vi "TranReport.vi"(0 "Rings":picture, 1 "3D Surface":refnum<vi>, 2 "annuli list":string[](array[string]), 5 "Output Cluster":T1 {"?" format="%.2f"; "?"."Y[i]=X[i]/Max|X|" format="%.2f"; "?"."output" format="%.2f"; "?" format="%.2f"; "?"."Y[i]=X[i]/Max|X|" format="%.2f"; "?"."?" format="%.2f"}, 7 "Trans Geometry":T2={"Radius (cm)"=9.0, "a (cm)"=4.0, "focus location"=9.0} {"focus location" format="%.2f"; "a (cm)" format="%.2f"; "Radius (cm)" format="%.2f"}, 9 "Center Hole":dbl format="%.2f", 11 "Variables":T3={"Number of rings"=1, "sound spd (cm/s)"=150000, "z span (cm)"=4.0, "z steps"=20, "y spacing (cm)"=0.01, "y steps"=50, "time step (s)"=1e-08, "z"=0.0, "y"=0.0, "ref delay"=0.0, "freq (MHz)"=4.71, "cycles"=300} {"freq (MHz)" format="%.2f"; "z span (cm)" format="%.2f"; "y" format="%.2f"; "ref delay" format="%.2f"; "y spacing (cm)" format="%.3f"; "z" format="%.2f"; "time step (s)" format="%.2e"}, 12 "case":bool, 13 "ring locations":string) -> ()   [LabVIEW 2022 SP3]
uses:
  <vilib>/Utility/NIReport.llb/Append Report Text (str wrap).vi
  <vilib>/Utility/NIReport.llb/NI_report.lvclass
panel:
  out "lateral pressure":cluster{"output":dbl[], "output":dbl[]}(graph)
  out "axial pressure":cluster{dbl[], "output":dbl[]}(graph)
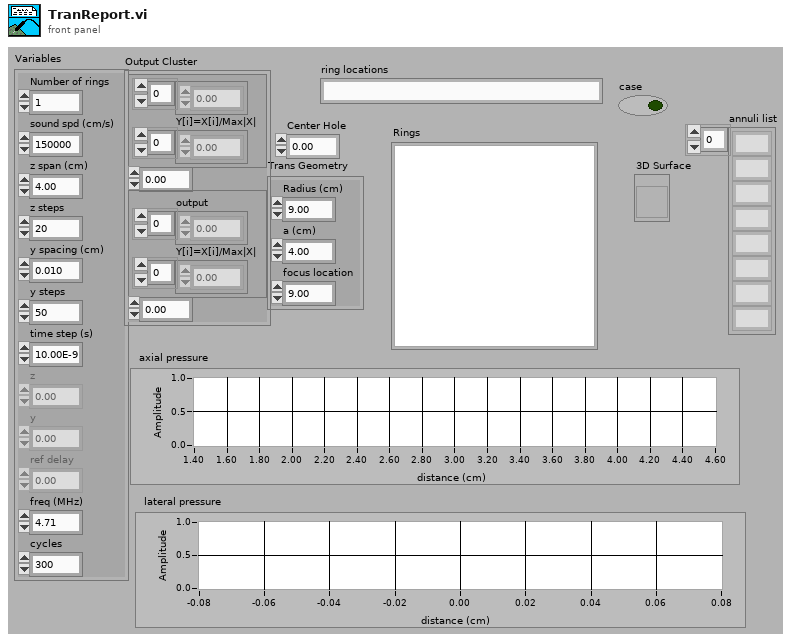
[diagram p1: front panel]
types:
  T1 = cluster{cluster{dbl[], "Y[i]=X[i]/Max|X|":dbl[]}, dbl, cluster{"output":dbl[], "Y[i]=X[i]/Max|X|":dbl[]}, dbl}
  T2 = cluster{"Radius (cm)":dbl, "a (cm)":dbl, "focus location":dbl}
  T3 = cluster{"Number of rings":i32, "sound spd (cm/s)":i32, "z span (cm)":dbl, "z steps":i32, "y spacing (cm)":dbl, "y steps":i32, "time step (s)":sgl, "z":dbl, "y":dbl, "ref delay":dbl, "freq (MHz)":dbl, "cycles":i32}
  T4 = cluster{"top":dbl, "left":dbl, "right":dbl, "bottom":dbl}
  T5 = cluster{"Italic":enum16{"Italic Unchanged", "Italic On", "Italic Off"}, "Strike Through":enum16{"Strike Through Unchanged", "Strike Through On", "Strike Through Off"}, "Underline":enum16{"Underline Unchanged", "Underline On", "Underline Off"}, "Bold":enum16{"Bold Unchanged", "Bold On", "Bold Off"}}
  T6 = cluster{"Charset (-1)":i16, "Weight (-1)":i16, "Name":string, "Size":string}
  T7 = cluster{"output":dbl[], "Y[i]=X[i]/Max|X|":dbl[]}
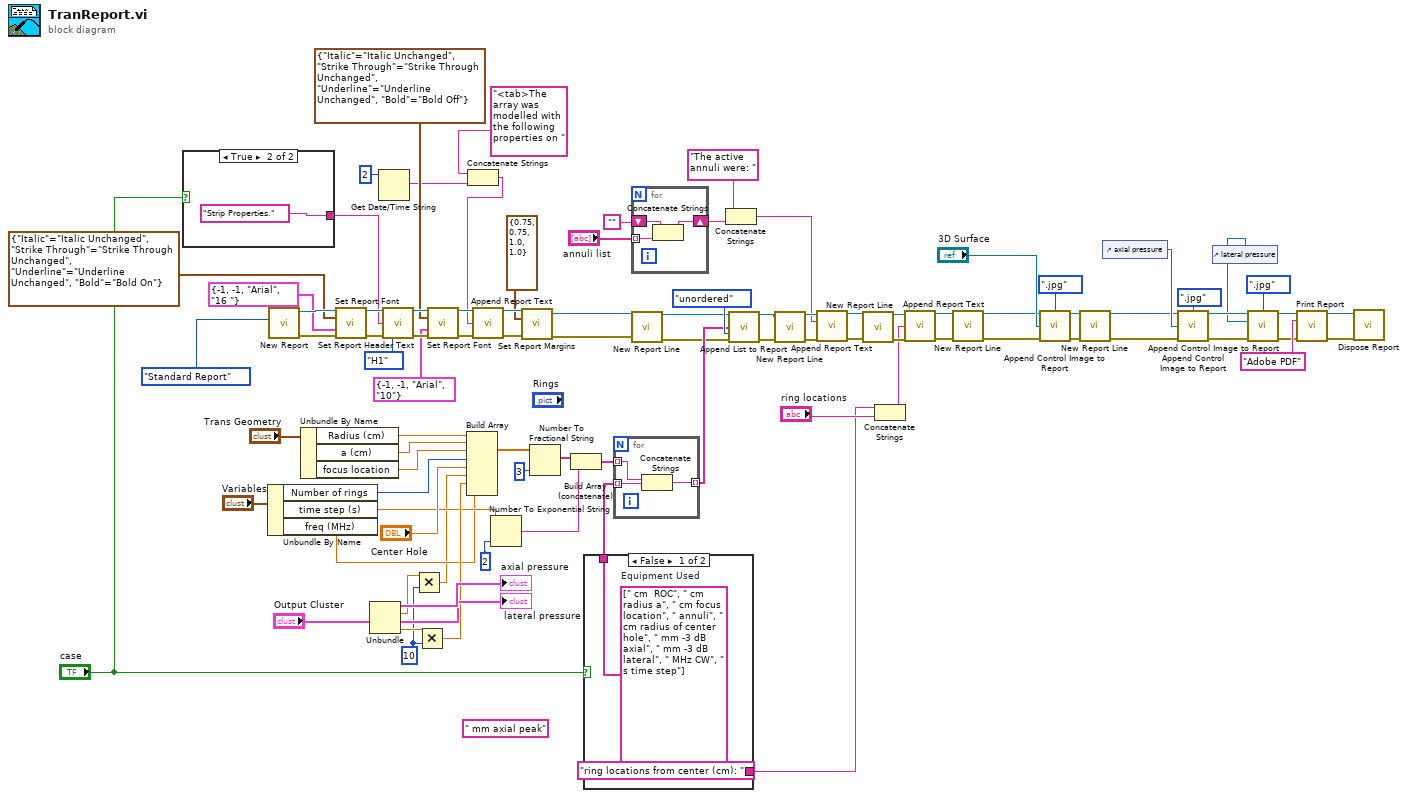
[diagram p0: block diagram]
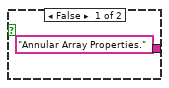
[diagram p2: hidden frame]
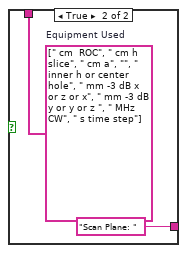
[diagram p3: hidden frame]
diagram:
  (unwired) " mm axial peak"
  w1 = 10
  n1 = case shown="True" "case" {
    tunnel: ["Annular Array Properties." ("Report Title") "Strip Properties." ("Report Title")] -> w49
    frame False {
    }
    frame True {
    }
  }
  n2 = Unbundle By Name("Variables") -> ("Number of rings"=w64:i32, "time step (s)"=w28:sgl, "freq (MHz)"=w14:dbl)
  n3 = call <vilib>:"New Report.vi"("report type"=enum16{"Standard Report", "HTML"}."Standard Report" ("Report Type")) -> ("report out"=w84:refnum<class "NI_report.lvclass">, "error out"=w83:errorcluster)  [unwired: 5 in, 8 out]
  n4 = Unbundle By Name("Trans Geometry") -> ("Radius (cm)"=w68:dbl, "a (cm)"=w67:dbl, "focus location"=w66:dbl)
  n5 = call-dynamic "Set Report Font.vi"("report in"=w84, "text options"=T5 {"Italic"=enum."Italic Unchanged", "Strike Through"=enum."Strike Through Unchanged", "Underline"=enum."Underline Unchanged", "Bold"=enum."Bold On"}, "font settings"=T6 {"Charset (-1)"=-1, "Weight (-1)"=-1, "Name"="Arial", "Size"="16 "}, "error in (no error)"=w83) -> ("report out"=w76:refnum<class "NI_report.lvclass">, "error out"=w77:errorcluster)  [unwired: 2 in, 8 out]
  n6 = Unbundle("Output Cluster") -> (→"axial pressure":cluster{dbl[], "Y[i]=X[i]/Max|X|":dbl[]}, w3:dbl, →"lateral pressure":T7, w39:dbl)
  n7 = Get Date/Time String(date format (0)=2) -> (date string=w6:string)  [unwired: 3 out]
  n8 = call-dynamic "Set Report Header Text.vi"("report in"=w76, "center header text"=w49, "error in (no error)"=w77, "HTML header size"=enum16{"H1", "H2", "H3", "H4", "H5", "H6", "H7"}."H1") -> ("report out"=w79:refnum<class "NI_report.lvclass">, "error out"=w80:errorcluster)  [unwired: 3 in, 7 out]
  n9 = Multiply(x=w3, y=w1) -> (x*y=w2:dbl)
  n10 = Multiply(x=w39, y=w1) -> (x*y=w38:dbl)
  n11 = call-dynamic "Set Report Font.vi"("report in"=w79, "text options"=T5 {"Italic"=enum."Italic Unchanged", "Strike Through"=enum."Strike Through Unchanged", "Underline"=enum."Underline Unchanged", "Bold"=enum."Bold Off"}, "font settings"=T6 {"Charset (-1)"=-1, "Weight (-1)"=-1, "Name"="Arial", "Size"="10"}, "error in (no error)"=w80) -> ("report out"=w82:refnum<class "NI_report.lvclass">, "error out"=w81:errorcluster)  [unwired: 2 in, 8 out]
  n12 = Build Array(w68, w67, w66, w64, "Center Hole", w2, w38, w14) -> (w62:dbl[])
  n13 = Concatenate Strings("<tab>The  array was modelled with the following properties on " ("Report text"), w6) -> (w5:string)
  n14 = call-poly <vilib>:"Append Report Text.vi"("report in"=w82, "text"=w5, "error in (no error)"=w81) -> ("report out"=w54:refnum<class "NI_report.lvclass">, "error out"=w53:errorcluster)  [unwired: 3 in, 8 out]
  n15 = Number To Exponential String(number=w28, precision (6)=2) -> (E-format string=w24:string)  [unwired: 2 out]
  n16 = call-dynamic "Set Report Margins.vi"("report in"=w54, "margins (1.00)"=T4 {"top"=0.75, "left"=0.75, "right"=1.0, "bottom"=1.0}, "error in (no error)"=w53) -> ("report out"=w51:refnum<class "NI_report.lvclass">, "error out"=w52:errorcluster)  [unwired: 1 in, 10 out]
  n17 = Number To Fractional String(number=w62, precision (6)=3) -> (F-format string=w26:string[])  [unwired: 2 out]
  n18 = Build Array (concatenate)(w26, w24) -> (w25:string[])
  n19 = case shown="False" "case" {
    tunnel: [w94 w96] -> w61
    tunnel: ["ring locations from center (cm): " "Scan Plane: "] -> w8
    frame False {
      w94 = string[] [" cm  ROC", " cm radius a", " cm focus location", " annuli", " cm radius of center hole", " mm -3 dB axial", " mm -3 dB lateral", " MHz CW", " s time step"]  # Equipment Used
    }
    frame True {
      w96 = string[] [" cm  ROC", " cm h slice", " cm a", "", " inner h or center hole", " mm -3 dB x or z or x", " mm -3 dB y or y or z ", " MHz CW", " s time step"]  # Equipment Used
    }
  }
  n20 = for {
    tunnel: w61 -> [w98] mode=indexing
    tunnel: w25 -> [w99] mode=indexing
    tunnel: [w97] -> w60 mode=indexing
    n21 = Concatenate Strings(w99, w98) -> (w97:string)
  }
  n22 = for {
    shift-right: [w102] -> w30
    shift-left: "" -> [w101]
    tunnel: "annuli list" -> [w100] mode=indexing
    n23 = Concatenate Strings(w101, w100) -> (w102:string)
  }
  n24 = call-dynamic "New Report Line.vi"("report in"=w51, "error in (no error)"=w52) -> ("report out"=w56:refnum<class "NI_report.lvclass">, "error out"=w55:errorcluster)  [unwired: 1 in, 11 out]
  n25 = Concatenate Strings("The active annuli were: " ("Report text"), w30) -> (w29:string)
  n26 = call-dynamic "Append List to Report.vi"("report in"=w56, "list elements"=w60, "list type (ordered)"=enum16{"unordered", "ordered"}."unordered", "error in (no error)"=w55) -> ("report out"=w37:refnum<class "NI_report.lvclass">, "error out"=w36:errorcluster)  [unwired: 4 in, 6 out]
  n27 = call-dynamic "New Report Line.vi"("report in"=w37, "error in (no error)"=w36) -> ("report out"=w35:refnum<class "NI_report.lvclass">, "error out"=w34:errorcluster)  [unwired: 1 in, 11 out]
  n28 = call-poly <vilib>:"Append Report Text.vi"("report in"=w35, "text"=w29, "error in (no error)"=w34) -> ("report out"=w20:refnum<class "NI_report.lvclass">, "error out"=w19:errorcluster)  [unwired: 3 in, 8 out]
  n29 = call-dynamic "New Report Line.vi"("report in"=w20, "error in (no error)"=w19) -> ("report out"=w18:refnum<class "NI_report.lvclass">, "error out"=w21:errorcluster)  [unwired: 1 in, 11 out]
  n30 = Concatenate Strings(w8, "ring locations") -> (w15:string)
  n31 = call-poly <vilib>:"Append Report Text.vi"("report in"=w18, "text"=w15, "error in (no error)"=w21) -> ("report out"=w17:refnum<class "NI_report.lvclass">, "error out"=w16:errorcluster)  [unwired: 3 in, 8 out]
  n32 = call-dynamic "New Report Line.vi"("report in"=w17, "error in (no error)"=w16) -> ("report out"=w13:refnum<class "NI_report.lvclass">, "error out"=w12:errorcluster)  [unwired: 1 in, 11 out]
  n33 = call-dynamic "Append Control Image to Report.vi"("report in"=w13, "image file type (.jpg)"=enum16{".jpg", ".png"}.".jpg" ("image file type(.png)"), "ctrl reference"="3D Surface", "error in (no error)"=w12) -> ("report out"=w86:refnum<class "NI_report.lvclass">, "error out"=w85:errorcluster)  [unwired: 4 in, 6 out]
  n34 = call-dynamic "New Report Line.vi"("report in"=w86, "error in (no error)"=w85) -> ("report out"=w11:refnum<class "NI_report.lvclass">, "error out"=w10:errorcluster)  [unwired: 1 in, 11 out]
  n35 = control-ref of="axial pressure"() -> (w23:refnum<vi>)
  n36 = call-dynamic "Append Control Image to Report.vi"("report in"=w11, "image file type (.jpg)"=enum16{".jpg", ".png"}.".jpg" ("image file type(.png)"), "ctrl reference"=w23, "error in (no error)"=w10) -> ("report out"=w58:refnum<class "NI_report.lvclass">, "error out"=w57:errorcluster)  [unwired: 4 in, 6 out]
  n37 = control-ref of="lateral pressure"() -> (w48:refnum<vi>)
  n38 = call-dynamic "Append Control Image to Report.vi"("report in"=w58, "image file type (.jpg)"=enum16{".jpg", ".png"}.".jpg" ("image file type(.png)"), "ctrl reference"=w48, "error in (no error)"=w57) -> ("report out"=w41:refnum<class "NI_report.lvclass">, "error out"=w40:errorcluster)  [unwired: 4 in, 6 out]
  n39 = call-dynamic "Print Report.vi"("report in"=w41, "printer name (default)"="Adobe PDF", "error in (no error)"=w40) -> ("report out"=w89:refnum<class "NI_report.lvclass">, "error out"=w90:errorcluster)  [unwired: 1 in, 10 out]
  n40 = call-dynamic "Dispose Report.vi"("report in"=w89, "error in (no error)"=w90) -> ()  [unwired: 3 in, 11 out]
